vi "SP Convert 1.5 to 2.0.vi"(1 "S Parameter 1.5 Test Parameters":T2={"Tag"="", "Calibration"=enum."Not Calibrated", "Stimulus"={"Use Instrument Settings"=FALSE, "Sweep Type"=enum."Linear", "Sweep"=[], "Blank Frequencies"=FALSE, "Power, dBm"=0.0, "IFBW, Hz"=0.0, "Sweep Time, s"=0.0}, "Measurements"=[], "Reports"={"Reports to Generate"=[], "Print Reports"=TRUE}, "Quick Mode"=FALSE} {"Stimulus"."Sweep Time, s" format="%.3g"; "Measurements"."Channel (CH 1)" items=["CH 1", "CH 2", "CH 3", "CH 4"]}) -> (0 "S Parameter 2.0 Test Parameters":T1={"Tag"="", "Stimulus"={"Use Instrument Settings"=FALSE, "Sweep Type"=enum."Linear", "Sweep"=[{"Fstart, MHz"=500.0, "Fstop, MHz"=1500.0, "Points"=201}], "Blank Frequencies"=FALSE, "Power, dBm"=999.0, "IFBW, Hz"=-1.0, "Sweep Time, s"=-1.0}, "Measurements"=[], "Reports"={"Reports to Generate"=[], "Print Reports"=FALSE}, "Quick Mode"=FALSE, "Display"={"Retain Settings"=TRUE, "Lock Control"=FALSE, "Plot Orientation"=enum."Single", "CH Controls"=[{"Trace Orientation"=enum."Overlay", "Frequency"={"Start"=500.0, "Stop"=1500.0, "Units"="MHz"}, "CH1Control"={"ChOn"=TRUE, "Measure"=0, "Format"=6, "Autoscale"=FALSE, "Reference"=0.0, "\nRefUnit"="dB/Div", "Position"=5.0, "Scale"=1.0, "ScaleUnit"="dB/Div", "LimitOn"=TRUE, "LimitFill"=FALSE, "Display Data"=0}, "CH2Control"={"ChOn"=TRUE, "Measure"=0, "Format"=6, "Autoscale"=FALSE, "Reference"=0.0, "\nRefUnit"="dB/Div", "Position"=5.0, "Scale"=1.0, "ScaleUnit"="dB/Div", "LimitOn"=TRUE, "LimitFill"=FALSE, "Display Data"=0}}, {"Trace Orientation"=enum."Overlay", "Frequency"={"Start"=500.0, "Stop"=1500.0, "Units"="MHz"}, "CH1Control"={"ChOn"=TRUE, "Measure"=0, "Format"=6, "Autoscale"=TRUE, "Reference"=0.0, "\nRefUnit"="dB/Div", "Position"=5.0, "Scale"=1.0, "ScaleUnit"="dB/Div", "LimitOn"=TRUE, "LimitFill"=FALSE, "Display Data"=0}, "CH2Control"={"ChOn"=TRUE, "Measure"=1, "Format"=0, "Autoscale"=TRUE, "Reference"=0.0, "\nRefUnit"="dB/Div", "Position"=5.0, "Scale"=1.0, "ScaleUnit"="dB/Div", "LimitOn"=TRUE, "LimitFill"=FALSE, "Display Data"=0}}, {"Trace Orientation"=enum."Overlay", "Frequency"={"Start"=500.0, "Stop"=1500.0, "Units"="MHz"}, "CH1Control"={"ChOn"=TRUE, "Measure"=0, "Format"=6, "Autoscale"=TRUE, "Reference"=0.0, "\nRefUnit"="dB/Div", "Position"=5.0, "Scale"=1.0, "ScaleUnit"="dB/Div", "LimitOn"=TRUE, "LimitFill"=FALSE, "Display Data"=0}, "CH2Control"={"ChOn"=TRUE, "Measure"=1, "Format"=0, "Autoscale"=TRUE, "Reference"=0.0, "\nRefUnit"="dB/Div", "Position"=5.0, "Scale"=1.0, "ScaleUnit"="dB/Div", "LimitOn"=TRUE, "LimitFill"=FALSE, "Display Data"=0}}, {"Trace Orientation"=enum."Overlay", "Frequency"={"Start"=500.0, "Stop"=1500.0, "Units"="MHz"}, "CH1Control"={"ChOn"=TRUE, "Measure"=0, "Format"=6, "Autoscale"=TRUE, "Reference"=0.0, "\nRefUnit"="dB/Div", "Position"=5.0, "Scale"=1.0, "ScaleUnit"="dB/Div", "LimitOn"=TRUE, "LimitFill"=FALSE, "Display Data"=0}, "CH2Control"={"ChOn"=TRUE, "Measure"=1, "Format"=0, "Autoscale"=TRUE, "Reference"=0.0, "\nRefUnit"="dB/Div", "Position"=5.0, "Scale"=1.0, "ScaleUnit"="dB/Div", "LimitOn"=TRUE, "LimitFill"=FALSE, "Display Data"=0}}]}, "Calibrations"=[enum."Not Calibrated", enum."Not Calibrated", enum."Not Calibrated", enum."Not Calibrated"]} {"Display"."CH Controls"."Frequency"."Stop" format="%.3g"; "Display"."CH Controls"."Frequency"."Start" format="%.3g"; "Display"."CH Controls"."CH2Control"."Reference" format="%#.2g"; "Display"."CH Controls"."CH2Control"."Display Data" items=["Data", "Memory", "Data/Memory"]; "Display"."CH Controls"."CH2Control"."Measure" items=["S11", "S21", "S12", "S22"]; "Display"."CH Controls"."CH2Control"."Format" items=["Log Mag", "Phase", "Delay", "Smith", "Polar", "Lin Mag", "SWR", "Loss", "Real", "Imaginary"]; "Display"."CH Controls"."CH2Control"."Scale" min=0.001 step=1.0 format="%#.2g"; "Display"."CH Controls"."CH2Control"."Position" min=0.0 max=10.0; "Display"."CH Controls"."CH1Control"."Reference" format="%#.2g"; "Display"."CH Controls"."CH1Control"."Display Data" items=["Data", "Memory", "Data/Memory"]; "Display"."CH Controls"."CH1Control"."Measure" items=["S11", "S21", "S12", "S22"]; "Display"."CH Controls"."CH1Control"."Format" items=["Log Mag", "Phase", "Delay", "Smith", "Polar", "Lin Mag", "SWR", "Loss", "Real", "Imaginary"]; "Display"."CH Controls"."CH1Control"."Scale" min=0.001 step=1.0 format="%#.2g"; "Display"."CH Controls"."CH1Control"."Position" min=0.0 max=10.0; "Stimulus"."Sweep Time, s" format="%.3g"; "Measurements"."Channel" min=1 max=99 step=1})   [LabVIEW 2011]
uses:
  TypeDefs/SP Test Parameters v1.5.ctl
  TypeDefs/SP Test Parameters v2.0.ctl
panel:
  # "Div"
  # "Div"
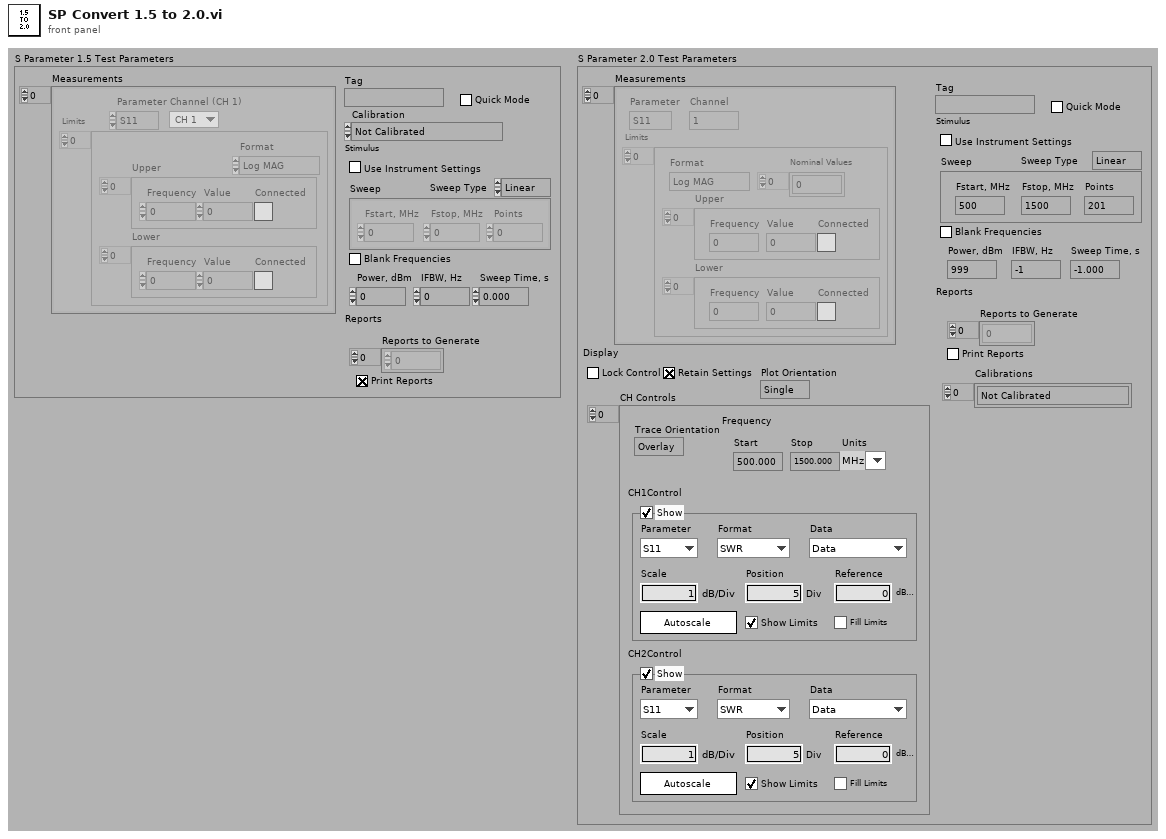
[diagram p1: front panel]
types:
  T1 = typedef "SP Test Parameters v2.0.ctl" = cluster{"Tag":string, "Stimulus":cluster{"Use Instrument Settings":bool, "Sweep Type":enum32{"Linear", "Log", "List", "Power", "CW"}, "Sweep":cluster{"Fstart, MHz":dbl, "Fstop, MHz":dbl, "Points":i32}[], "Blank Frequencies":bool, "Power, dBm":dbl, "IFBW, Hz":dbl, "Sweep Time, s":dbl}, "Measurements":cluster{"Parameter":enum32{"S11", "S21", "S12", "S22"}, "Channel":i32, "Limits":cluster{"Format":enum16{"Log MAG", "Lin MAG", "VSWR", "Phase", "Delay", "Insertion Loss", "Isolation", "Return Loss"}, "Upper":cluster{"Frequency":dbl, "Value":dbl, "Connected":bool}[], "Lower":cluster{"Frequency":dbl, "Value":dbl, "Connected":bool}[], "Nominal Values":dbl[]}[]}[], "Reports":cluster{"Reports to Generate":i32[], "Print Reports":bool}, "Quick Mode":bool, "Display":cluster{"Retain Settings":bool, "Lock Control":bool, "Plot Orientation":enum32{"Single", "Dual", "Quad"}, "CH Controls":cluster{"Trace Orientation":enum32{"Overlay", "Split"}, "Frequency":cluster{"Start":dbl, "Stop":dbl, "Units":string}, "CH1Control":cluster{"ChOn":bool, "Measure":i32, "Format":i32, "Autoscale":bool, "Reference":dbl, "\nRefUnit":string, "Position":dbl, "Scale":dbl, "ScaleUnit":string, "LimitOn":bool, "LimitFill":bool, "Display Data":u16}, "CH2Control":cluster{"ChOn":bool, "Measure":i32, "Format":i32, "Autoscale":bool, "Reference":dbl, "\nRefUnit":string, "Position":dbl, "Scale":dbl, "ScaleUnit":string, "LimitOn":bool, "LimitFill":bool, "Display Data":u16}}[]}, "Calibrations":enum32{"Not Calibrated", "Response", "Response and Isolation", "Full 1-Port (Port 1)", "Full 1-Port (Port 2)", "Full 2-Port", "One Path 2-Port", "TRL/LRM  2-Port"}[]}
  T2 = typedef "SP Test Parameters v1.5.ctl" = cluster{"Tag":string, "Calibration":enum32{"Not Calibrated", "Response", "Response and Isolation", "Full 1-Port (Port 1)", "Full 1-Port (Port 2)", "Full 2-Port", "One Path 2-Port", "TRL/LRM  2-Port"}, "Stimulus":cluster{"Use Instrument Settings":bool, "Sweep Type":enum32{"Linear", "Log", "List", "Power", "CW"}, "Sweep":cluster{"Fstart, MHz":dbl, "Fstop, MHz":dbl, "Points":i32}[], "Blank Frequencies":bool, "Power, dBm":dbl, "IFBW, Hz":dbl, "Sweep Time, s":dbl}, "Measurements":cluster{"Parameter":enum32{"S11", "S21", "S12", "S22"}, "Limits":cluster{"Format":enum16{"Log MAG", "Lin MAG", "VSWR", "Phase", "Delay", "Insertion Loss", "Isolation", "Return Loss"}, "Upper":cluster{"Frequency":dbl, "Value":dbl, "Connected":bool}[], "Lower":cluster{"Frequency":dbl, "Value":dbl, "Connected":bool}[]}[], "Channel (CH 1)":u16}[], "Reports":cluster{"Reports to Generate":i32[], "Print Reports":bool}, "Quick Mode":bool}
  T3 = cluster{"Use Instrument Settings":bool, "Sweep Type":enum32{"Linear", "Log", "List", "Power", "CW"}, "Sweep":cluster{"Fstart, MHz":dbl, "Fstop, MHz":dbl, "Points":i32}[], "Blank Frequencies":bool, "Power, dBm":dbl, "IFBW, Hz":dbl, "Sweep Time, s":dbl}
  T4 = cluster{"Reports to Generate":i32[], "Print Reports":bool}
  T5 = enum32{"Not Calibrated", "Response", "Response and Isolation", "Full 1-Port (Port 1)", "Full 1-Port (Port 2)", "Full 2-Port", "One Path 2-Port", "TRL/LRM  2-Port"}
  T6 = cluster{"Parameter":enum32{"S11", "S21", "S12", "S22"}, "Limits":cluster{"Format":enum16{"Log MAG", "Lin MAG", "VSWR", "Phase", "Delay", "Insertion Loss", "Isolation", "Return Loss"}, "Upper":cluster{"Frequency":dbl, "Value":dbl, "Connected":bool}[], "Lower":cluster{"Frequency":dbl, "Value":dbl, "Connected":bool}[]}[], "Channel (CH 1)":u16}[]
  T7 = cluster{"Parameter":enum32{"S11", "S21", "S12", "S22"}, "Channel":i32, "Limits":cluster{"Format":enum16{"Log MAG", "Lin MAG", "VSWR", "Phase", "Delay", "Insertion Loss", "Isolation", "Return Loss"}, "Upper":cluster{"Frequency":dbl, "Value":dbl, "Connected":bool}[], "Lower":cluster{"Frequency":dbl, "Value":dbl, "Connected":bool}[], "Nominal Values":dbl[]}[]}[]
  T8 = cluster{"Parameter":enum32{"S11", "S21", "S12", "S22"}, "Channel":i32, "Limits":cluster{"Format":enum16{"Log MAG", "Lin MAG", "VSWR", "Phase", "Delay", "Insertion Loss", "Isolation", "Return Loss"}, "Upper":cluster{"Frequency":dbl, "Value":dbl, "Connected":bool}[], "Lower":cluster{"Frequency":dbl, "Value":dbl, "Connected":bool}[], "Nominal Values":dbl[]}[]}
  T9 = cluster{"Format":enum16{"Log MAG", "Lin MAG", "VSWR", "Phase", "Delay", "Insertion Loss", "Isolation", "Return Loss"}, "Upper":cluster{"Frequency":dbl, "Value":dbl, "Connected":bool}[], "Lower":cluster{"Frequency":dbl, "Value":dbl, "Connected":bool}[], "Nominal Values":dbl[]}[]
  T10 = enum32{"Not Calibrated", "Response", "Response and Isolation", "Full 1-Port (Port 1)", "Full 1-Port (Port 2)", "Full 2-Port", "One Path 2-Port", "TRL/LRM  2-Port"}[]
  T11 = cluster{"Format":enum16{"Log MAG", "Lin MAG", "VSWR", "Phase", "Delay", "Insertion Loss", "Isolation", "Return Loss"}, "Upper":cluster{"Frequency":dbl, "Value":dbl, "Connected":bool}[], "Lower":cluster{"Frequency":dbl, "Value":dbl, "Connected":bool}[], "Nominal Values":dbl[]}
  T12 = cluster{"Format":enum16{"Log MAG", "Lin MAG", "VSWR", "Phase", "Delay", "Insertion Loss", "Isolation", "Return Loss"}, "Upper":cluster{"Frequency":dbl, "Value":dbl, "Connected":bool}[], "Lower":cluster{"Frequency":dbl, "Value":dbl, "Connected":bool}[]}[]
  T13 = enum16{"Log MAG", "Lin MAG", "VSWR", "Phase", "Delay", "Insertion Loss", "Isolation", "Return Loss"}
  T14 = cluster{"Frequency":dbl, "Value":dbl, "Connected":bool}[]
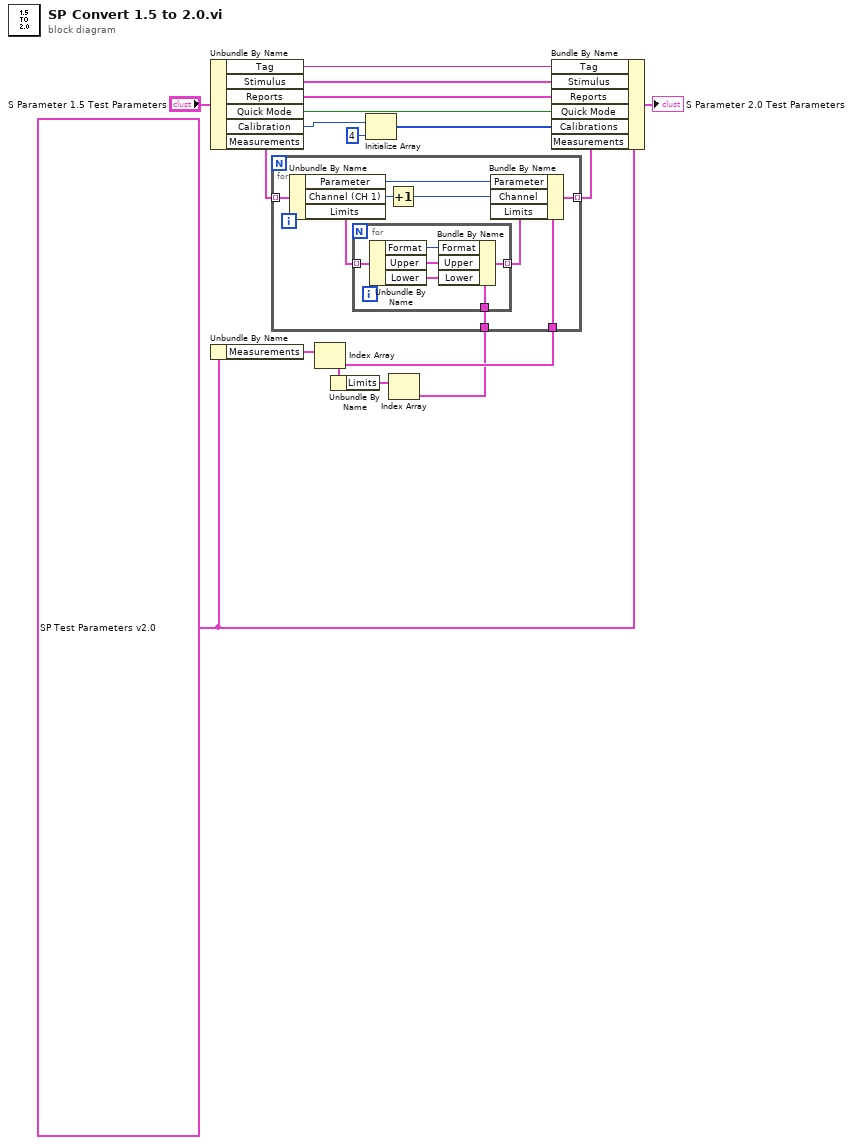
[diagram p0: block diagram]
diagram:
  w3 = T1 {"Tag"="", "Stimulus"={"Use Instrument Settings"=FALSE, "Sweep Type"=enum."Linear", "Sweep"=[{"Fstart, MHz"=500.0, "Fstop, MHz"=1500.0, "Points"=201}], "Blank Frequencies"=FALSE, "Power, dBm"=999.0, "IFBW, Hz"=-1.0, "Sweep Time, s"=-1.0}, "Measurements"=[{"Parameter"=enum."S11", "Channel"=1, "Limits"=[]}, {"Parameter"=enum."S21", "Channel"=2, "Limits"=[]}], "Reports"={"Reports to Generate"=[], "Print Reports"=FALSE}, "Quick Mode"=FALSE, "Display"={"Retain Settings"=TRUE, "Lock Control"=FALSE, "Plot Orientation"=enum."Single", "CH Controls"=[{"Trace Orientation"=enum."Overlay", "Frequency"={"Start"=500.0, "Stop"=1500.0, "Units"="MHz"}, "CH1Control"={"ChOn"=TRUE, "Measure"=0, "Format"=0, "Autoscale"=TRUE, "Reference"=0.0, "\nRefUnit"="dB/Div", "Position"=5.0, "Scale"=10.0, "ScaleUnit"="dB/Div", "LimitOn"=TRUE, "LimitFill"=FALSE, "Display Data"=0}, "CH2Control"={"ChOn"=TRUE, "Measure"=1, "Format"=0, "Autoscale"=TRUE, "Reference"=0.0, "\nRefUnit"="dB/Div", "Position"=5.0, "Scale"=10.0, "ScaleUnit"="dB/Div", "LimitOn"=TRUE, "LimitFill"=FALSE, "Display Data"=0}}, {"Trace Orientation"=enum."Overlay", "Frequency"={"Start"=500.0, "Stop"=1500.0, "Units"="MHz"}, "CH1Control"={"ChOn"=TRUE, "Measure"=0, "Format"=0, "Autoscale"=TRUE, "Reference"=0.0, "\nRefUnit"="dB/Div", "Position"=5.0, "Scale"=10.0, "ScaleUnit"="dB/Div", "LimitOn"=TRUE, "LimitFill"=FALSE, "Display Data"=0}, "CH2Control"={"ChOn"=TRUE, "Measure"=0, "Format"=0, "Autoscale"=TRUE, "Reference"=0.0, "\nRefUnit"="dB/Div", "Position"=5.0, "Scale"=10.0, "ScaleUnit"="dB/Div", "LimitOn"=TRUE, "LimitFill"=FALSE, "Display Data"=0}}, {"Trace Orientation"=enum."Overlay", "Frequency"={"Start"=500.0, "Stop"=1500.0, "Units"="MHz"}, "CH1Control"={"ChOn"=TRUE, "Measure"=0, "Format"=0, "Autoscale"=TRUE, "Reference"=0.0, "\nRefUnit"="dB/Div", "Position"=5.0, "Scale"=10.0, "ScaleUnit"="dB/Div", "LimitOn"=TRUE, "LimitFill"=FALSE, "Display Data"=0}, "CH2Control"={"ChOn"=TRUE, "Measure"=0, "Format"=0, "Autoscale"=TRUE, "Reference"=0.0, "\nRefUnit"="dB/Div", "Position"=5.0, "Scale"=10.0, "ScaleUnit"="dB/Div", "LimitOn"=TRUE, "LimitFill"=FALSE, "Display Data"=0}}, {"Trace Orientation"=enum."Overlay", "Frequency"={"Start"=500.0, "Stop"=1500.0, "Units"="MHz"}, "CH1Control"={"ChOn"=TRUE, "Measure"=0, "Format"=0, "Autoscale"=TRUE, "Reference"=0.0, "\nRefUnit"="dB/Div", "Position"=5.0, "Scale"=10.0, "ScaleUnit"="dB/Div", "LimitOn"=TRUE, "LimitFill"=FALSE, "Display Data"=0}, "CH2Control"={"ChOn"=TRUE, "Measure"=0, "Format"=0, "Autoscale"=TRUE, "Reference"=0.0, "\nRefUnit"="dB/Div", "Position"=5.0, "Scale"=10.0, "ScaleUnit"="dB/Div", "LimitOn"=TRUE, "LimitFill"=FALSE, "Display Data"=0}}]}, "Calibrations"=[enum."Not Calibrated", enum."Not Calibrated", enum."Not Calibrated", enum."Not Calibrated"]} ("S Parameter Test Parameters")
  n1 = Unbundle By Name("S Parameter 1.5 Test Parameters") -> ("Tag"=w16:string, "Stimulus"=w10:T3, "Reports"=w11:T4, "Quick Mode"=w12:bool, "Calibration"=w8:T5, "Measurements"=w15:T6)
  n2 = Unbundle By Name(w3) -> ("Measurements"=w13:T7)
  n3 = Index Array(array=w13) -> (element=w6:T8)  [unwired: 1 in]
  n4 = Unbundle By Name(w6) -> ("Limits"=w5:T9)
  n5 = Initialize Array(w8, 4) -> (w7:T10)
  n6 = Index Array(array=w5) -> (element=w4:T11)  [unwired: 1 in]
  n7 = for {
    tunnel: w15 -> [w25] mode=indexing
    tunnel: w6 -> [w24]
    tunnel: [w22] -> w14 mode=indexing
    tunnel: w4 -> [w18]
    n8 = Unbundle By Name(w25) -> ("Parameter"=w23:enum32{"S11", "S21", "S12", "S22"}, "Channel (CH 1)"=w21:u16, "Limits"=w19:T12)
    n9 = for {
      tunnel: w19 -> [w31] mode=indexing
      tunnel: w18 -> [w30]
      tunnel: [w26] -> w17 mode=indexing
      n10 = Unbundle By Name(w31) -> ("Format"=w27:T13, "Upper"=w28:T14, "Lower"=w29:T14)
      n11 = Bundle By Name(cluster=w30, "Format"=w27, "Upper"=w28, "Lower"=w29) -> (w26:T11)
    }
    n12 = Increment(x=w21) -> (x+1=w20:u16)
    n13 = Bundle By Name(cluster=w24, "Parameter"=w23, "Channel"=w20, "Limits"=w17) -> (w22:T8)
  }
  n14 = Bundle By Name(cluster=w3, "Tag"=w16, "Stimulus"=w10, "Reports"=w11, "Quick Mode"=w12, "Calibrations"=w7, "Measurements"=w14) -> (→"S Parameter 2.0 Test Parameters":T1)
